vi "PID Derivative Action Buffered (DBL Array).vi"(5 "Kd":dbl[](array[numeric]) format="%.2f", 6 "initialize (F)":bool, 7 "process variable":dbl[](array[numeric]) format="%.2f", 8 "dt (min)":dbl format="%.3f", 10 "previous  process variable":dbl[](array[numeric]), 11 "previous derivative action":dbl[](array[numeric])) -> (2 "process variable buffer":dbl[](array[numeric]), 3 "derivative action":dbl[](array[numeric]) format="%.2f")   [LabVIEW 2020, in "NI_PID_pid.lvlib"]
uses:
  NI_PID_pid.lvlib
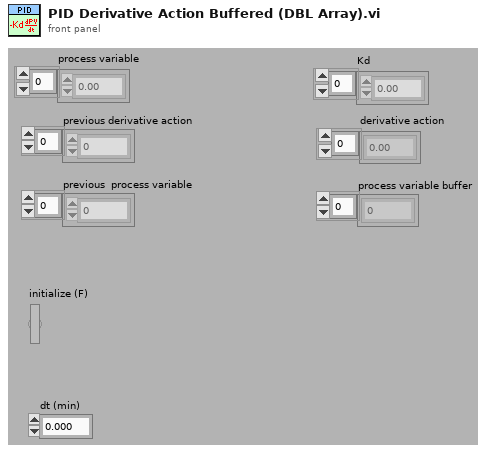
[diagram p1: front panel]
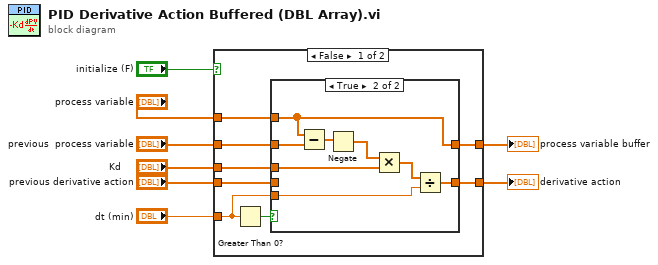
[diagram p0: block diagram]
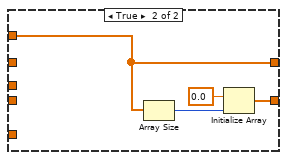
[diagram p3: hidden frame]
diagram:
  n1 = case shown="False" "initialize (F)" {
    tunnel: "previous  process variable" -> [w16 _]
    tunnel: "Kd" -> [w13 _]
    tunnel: "process variable" -> [w15 w30]
    tunnel: [w12 w30] -> w1
    tunnel: [w14 w28] -> w3
    tunnel: "previous derivative action" -> [w10 _]
    tunnel: "dt (min)" -> [w9 _]
    frame False {
      n2 = Greater Than 0?(x=w9) -> (x > 0?=w11:bool)
      n3 = case shown="True" w11 {
        tunnel: w16 -> [w18 w24]
        tunnel: w9 -> [_ w23]
        tunnel: w15 -> [_ w19]
        tunnel: [w17 w22] -> w14
        tunnel: w13 -> [_ w20]
        tunnel: [w18 w19] -> w12
        tunnel: w10 -> [w17 _]
        frame False {
          # "dt = 0 min"
        }
        frame True {
          n4 = Subtract(x=w19, y=w24) -> (x-y=w26:dbl[])
          n5 = Negate(x=w26) -> (-x=w21:dbl[])
          n6 = Multiply(x=w21, y=w20) -> (x*y=w25:dbl[])
          n7 = Divide(x=w25, y=w23) -> (x/y=w22:dbl[])
        }
      }
    }
    frame True {
      n8 = Array Size(array=w30) -> (size(s)=w29:i32)
      n9 = Initialize Array(0.0 ("Element Data"), w29) -> (w28:dbl[])
    }
  }
  "derivative action" <- w3
  "process variable buffer" <- w1
